vi "Util.Cmprs.LZW.CU.BitStream.Width__ogtk.vi"(9 "ImageBits":i32, 10 "Reset":i16, 11 "Code":i16) -> (2 "Bit Width next":i32, 3 "Bit Width":i32)   [LabVIEW 2012]
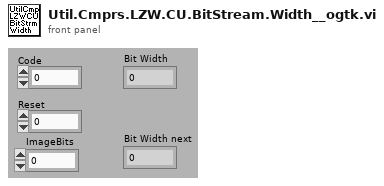
[diagram p1: front panel]
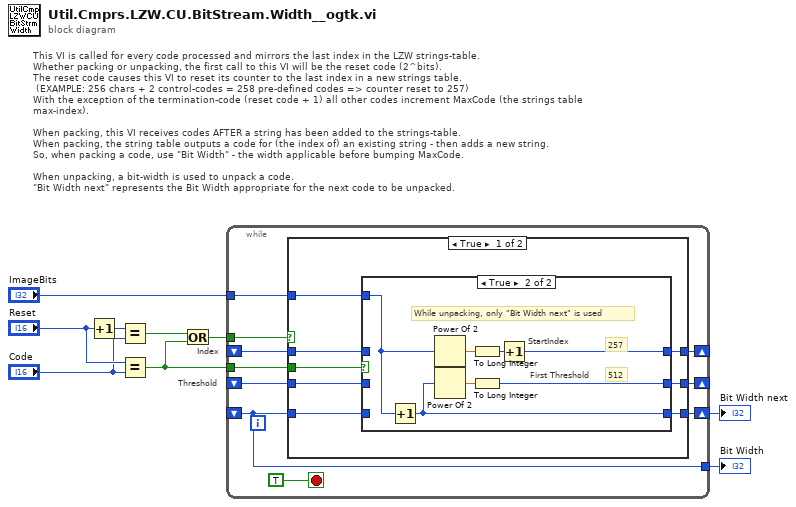
[diagram p0: block diagram]
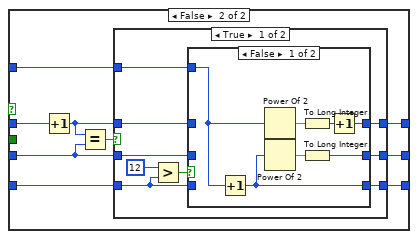
[diagram p3: hidden frame]
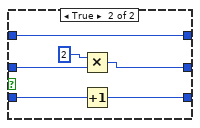
[diagram p4: hidden frame]
diagram:
  # "Threshold"
  # "Index"
  # "This VI is called for every code processed and mirrors the last index in the LZW strings-table.\nWhether packing or unpacking, the first call to this VI will be the reset code (2^bits).\nThe reset code causes this VI to reset its counter to the last index in a new strings table.\n (EXAMPLE: 256 chars + 2 control-codes = 258 pre-defined codes => counter reset to 257)\nWith the exception of the termination-code (reset code + 1) all other codes increment MaxCode (the strings table max-index).\n\nWhen packing, this VI receives codes AFTER a string has been added to the strings-table.\nWhen packing, the string table outputs a code for (the index of) an existing string - then adds a new string.\nSo, when packing a code, use \"Bit Width\" - the width applicable before bumping MaxCode.\n\nWhen unpacking, a bit-width is used to unpack a code.\n\"Bit Width next\" represents the Bit Width appropriate for the next code to be unpacked."
  n1 = Increment(x="Reset") -> (x+1=w4:i16)
  n2 = Equal?(x=w4, y="Code") -> (x = y?=w2:bool)
  n3 = Equal?(x="Reset", y="Code") -> (x = y?=w1:bool)
  n4 = Or(x=w2, y=w1) -> (x .or. y?=w3:bool)
  n5 = while {
    shift-right: [w19] -> _
    shift-left: _ -> [w16]
    shift-right: [w18] -> w8
    shift-left: _ -> [w15]
    tunnel: [w15] -> w9
    tunnel: "ImageBits" -> [w14]
    shift-right: [w13] -> _
    shift-left: _ -> [w12]
    tunnel: w3 -> [w11]
    tunnel: w1 -> [w10]
    stop <- TRUE stop-if-true
    n6 = case shown="True" w11 {
      tunnel: [w26 w45] -> w19
      tunnel: [w25 w43] -> w18
      tunnel: w15 -> [w21 w44]
      tunnel: w16 -> [w23 w46]
      tunnel: w14 -> [w27 w38]
      tunnel: [w24 w39] -> w13
      tunnel: w12 -> [w22 w40]
      tunnel: w10 -> [w20 _]
      frame True {
        n7 = case shown="True" w20 {
          tunnel: w27 -> [_ w34]
          tunnel: [w28 w33] -> w26
          tunnel: [w30 w32] -> w25
          tunnel: [w29 w31] -> w24
          tunnel: w23 -> [w28 _]
          tunnel: w22 -> [w29 _]
          tunnel: w21 -> [w30 _]
          frame False {
          }
          frame True {
            # "512"
            # "257"
            # "While unpacking, only \"Bit Width next\" is used"
            # "First Threshold"
            # "StartIndex"
            n8 = Increment(x=w34) -> (x+1=w32:i32)
            n9 = Power Of 2(x=w34) -> (2^x=w36:dbl)
            n10 = Power Of 2(x=w32) -> (2^x=w37:dbl)
            n11 = To Long Integer(number=w36) -> (32bit integer=w35:i32)
            n12 = To Long Integer(number=w37) -> (32bit integer=w31:i32)
            n13 = Increment(x=w35) -> (x+1=w33:i32)
          }
        }
      }
      frame False {
        n14 = Increment(x=w46) -> (x+1=w42:i32)
        n15 = Equal?(x=w42, y=w40) -> (x = y?=w41:bool)
        n16 = case shown="True" w41 {
          tunnel: w42 -> [w48 w71]
          tunnel: [w47 w71] -> w45
          tunnel: w44 -> [w49 w70]
          tunnel: [w50 w70] -> w43
          tunnel: w40 -> [w52 w69]
          tunnel: [w51 w69] -> w39
          tunnel: w38 -> [w55 _]
          frame True {
            n17 = Greater?(x=12, y=w49) -> (0:w53:bool)
            n18 = case shown="False" w53 {
              tunnel: w55 -> [w56 _]
              tunnel: w52 -> [_ w68]
              tunnel: [w57 w66] -> w51
              tunnel: [w60 w65] -> w50
              tunnel: w49 -> [_ w64]
              tunnel: w48 -> [_ w63]
              tunnel: [w59 w63] -> w47
              frame False {
                n19 = Increment(x=w56) -> (x+1=w60:i32)
                n20 = Power Of 2(x=w56) -> (2^x=w62:dbl)
                n21 = Power Of 2(x=w60) -> (2^x=w58:dbl)
                n22 = To Long Integer(number=w62) -> (32bit integer=w61:i32)
                n23 = To Long Integer(number=w58) -> (32bit integer=w57:i32)
                n24 = Increment(x=w61) -> (x+1=w59:i32)
              }
              frame True {
                n25 = Multiply(x=2 ("y"), y=w68) -> (x*y=w66:i32)
                n26 = Increment(x=w64) -> (x+1=w65:i32)
              }
            }
          }
          frame False {
          }
        }
      }
    }
  }
  "Bit Width" <- w9
  "Bit Width next" <- w8
